vi "Alternating_LEDs.vi"() -> ()   [LabVIEW 2015]
panel:
  in  "?":bool
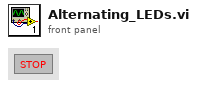
[diagram p1: front panel]
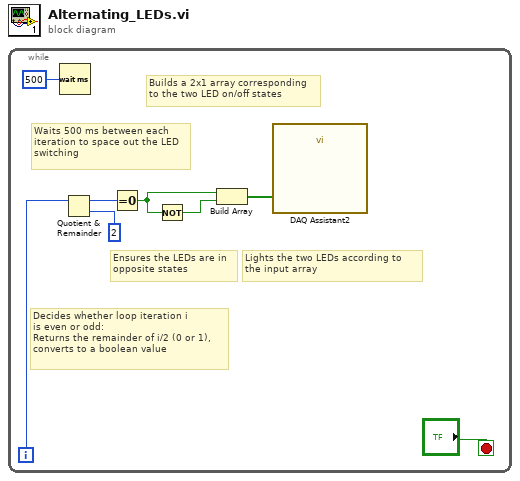
[diagram p0: block diagram]
diagram:
  n1 = while {
    i -> [w5]
    stop <- "?" stop-if-true
    # "Ensures the LEDs are in \nopposite states"
    # "Lights the two LEDs according to \nthe input array"
    # "Waits 500 ms between each \niteration to space out the LED\nswitching"
    # "Decides whether loop iteration i \nis even or odd: \nReturns the remainder of i/2 (0 or 1), \nconverts to a boolean value"
    # "Builds a 2x1 array corresponding\nto the two LED on/off states"
    n2 = Wait (ms)(milliseconds to wait=500) -> ()  [unwired: 1 out]
    n3 = Quotient & Remainder(x=w5, y=2) -> (x-y*floor(x/y)=w4:i32)  [unwired: 1 out]
    n4 = Equal To 0?(x=w4) -> (x = 0?=w3:bool)
    n5 = Not(x=w3) -> (.not. x?=w2:bool)
    n6 = Build Array(w3, w2) -> (w7:bool[])
    n7 = call "DAQ Assistant2"("data"=w7) -> ()  [unwired: 17 in, 2 out]
  }
